vi "start.vi"(8 "error in (no error)":errorcluster, 11 "HamegHMPSupply in":refnum<class "HamegHMPSupply.lvclass">) -> (0 "error out":errorcluster, 3 "HamegHMPSupply out":refnum<class "HamegHMPSupply.lvclass">)   [LabVIEW 2011, in "Hardware.lvlib" / "Channels.lvlib" / "HamegHMPSupply.lvclass"]
doc: "Abstract Method\n\nStarts/Arms the AnalogOutput task. Normally the AnalogOutput device is configured to wait for a trigger signal, therefore, in this case the method Arms the device ready for recieving its trigger upon which it will start outputing immediately its data."
uses:
  HamegHMPSupply.lvclass
  HamegHMPSupply.lvclass/HamegHMPSupply.ctl
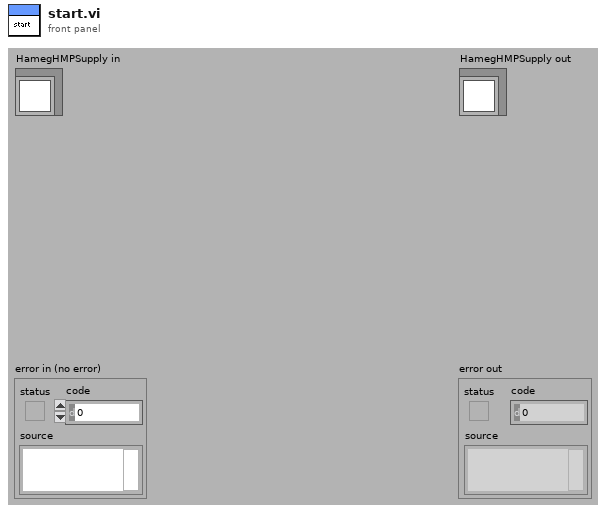
[diagram p1: front panel]
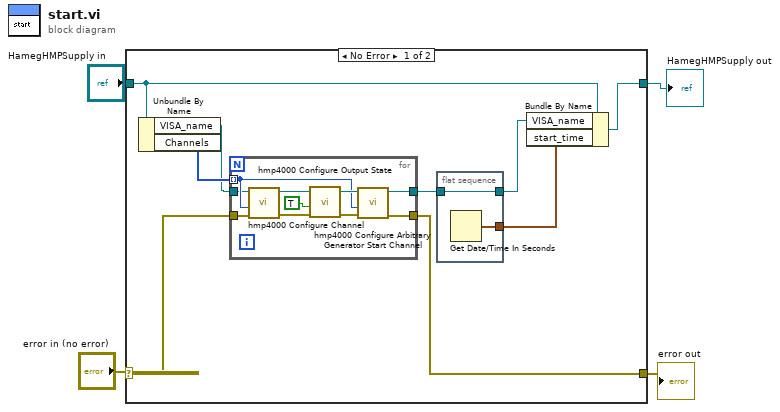
[diagram p0: block diagram]
diagram:
  n1 = case shown="No Error" "error in (no error)" {
    selector: "error in (no error)" -> [w8 w27]
    tunnel: [w11 w26] -> w3
    tunnel: "HamegHMPSupply in" -> [w12 w26]
    tunnel: [w13 w27] -> w1
    frame No Error {
      n2 = Unbundle By Name(w12) -> ("VISA_name"=w9:refnum<visa-resource-name>, "Channels"=w10:i32[])
      n3 = for {
        tunnel: w9 -> [w16]
        tunnel: w10 -> [w17] mode=indexing
        tunnel: w8 -> [w20]
        tunnel: [w25] -> w13
        tunnel: [w24] -> w7
        n4 = call <instrlib>:"hmp4000 Configure Channel.vi"("error in (no error)"=w20, "Channel (Channel 1)"=w17, "VISA resource name"=w16) -> ("error out"=w18:errorcluster, "VISA resource name out"=w19:refnum<visa-resource-name>)  [unwired: 7 in]
        n5 = call <instrlib>:"hmp4000 Configure Output State.vi"("error in (no error)"=w18, "Output State (Off)"=TRUE, "VISA resource name"=w19) -> ("error out"=w21:errorcluster, "VISA resource name out"=w22:refnum<visa-resource-name>)  [unwired: 7 in]
        n6 = call <instrlib>:"hmp4000 Configure Arbitrary Generator Start Channel.vi"("error in (no error)"=w21, "Channel (Channel 1)"=w17, "VISA resource name"=w22) -> ("error out"=w25:errorcluster, "VISA resource name out"=w24:refnum<visa-resource-name>)  [unwired: 7 in]
      }
      n7 = flat-sequence {
        tunnel: [w15] -> w6
        tunnel: w7 -> [w15]
        tunnel: [w14] -> w5
        frame #0 {
          n8 = Get Date/Time In Seconds() -> (seconds since 1Jan1904=w14:timestamp)
        }
      }
      n9 = Bundle By Name(cluster=w12, "VISA_name"=w6, "start_time"=w5) -> (w11:refnum<class "HamegHMPSupply.lvclass">)
    }
    frame Error {
    }
  }
  "error out" <- w1
  "HamegHMPSupply out" <- w3
